vi "GetExternalInterfaces.vi"(8 "ErrorIn":errorcluster, 11 "ObjectIn":refnum<class "YAFTAF.lvclass">) -> (0 "ErrorOut":errorcluster, 2 "ExternalInterfaces":T1[](array[typedef]), 3 "ObjectOut":refnum<class "YAFTAF.lvclass">)   [LabVIEW 2021, in "YAFTAF.lvclass"]
uses:
  YAFTAF.lvclass
  C:/Localdata/Projects/TriekselSoft/TriekselsoftApplicationFramework/Source/.Externals/Library_YAF/YActor/YActor.lvclass
  Library_TAF_Support/ClusterArrayConversion/BundledArray.ctl
  YActor/YActor.lvclass/YActor.ctl
  YActor/ExeCmd_sync.vi
  YActor/private/SendCommand.vi
  YActor/private/WaitForReply.vi
  YActor/private/CreateLocalVI.vi
  YActor/private/ExeuteInlineVI.vi
  YActor/private/GetRemoteVIRef.vi
  YActor/private/GetNameOfVI.vi
  YActor/QuickCast.vi
  YActor/private/VINameProperty.vi
  YActor/private/MessageCounter.vi
  YActor/InlineReferencePool.vi
  YActor/private/ExecuteVI.vi
  YActor/YActor.lvclass
  YAFTAF.lvclass/YAFTAF.ctl
  Library_TAF_Support/ClusterArrayConversion/ClusterArrayConversion.lvlib
  C:/Localdata/Projects/TriekselSoft/TriekselsoftApplicationFramework/Source/.Externals/Interface_UserInterface_IFrontPanel/IFrontPanel/IFrontPanel.lvclass
  C:/Localdata/Projects/TriekselSoft/TriekselsoftApplicationFramework/Source/IInterface/IInterface.lvclass
  C:/Localdata/Projects/TriekselSoft/TriekselsoftApplicationFramework/Source/.Externals/Interface_Object_ICreateDestroy/ICreateDestroy/ICreateDestroy.lvclass
  C:/Localdata/Projects/TriekselSoft/TriekselsoftApplicationFramework/Source/.Externals/Interface_Object_IPersistentData/IPersistentData/IPersistentData.lvclass
  C:/Localdata/Projects/TriekselSoft/TriekselsoftApplicationFramework/Source/.Externals/Interface_TAF_ITAFObject/ITAFObject/ITAFObject.lvclass
  C:/Localdata/Projects/TriekselSoft/TriekselsoftApplicationFramework/Source/.Externals/Library_YAF/YAFTAF/YAFTAF.lvclass
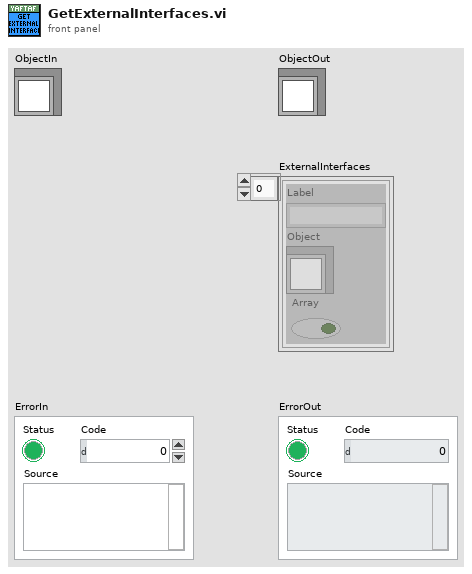
[diagram p1: front panel]
types:
  T1 = typedef "ClusterArrayConversion.lvlib/BundledArray.ctl" = cluster{"Label":string, "Object":refnum<class>, "Array":bool}
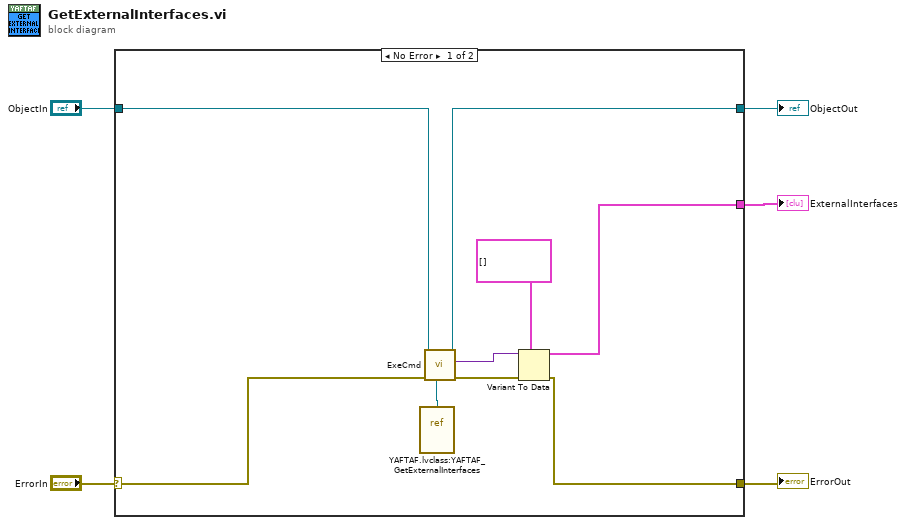
[diagram p0: block diagram]
diagram:
  n1 = case shown="No Error" "ErrorIn" {
    selector: "ErrorIn" -> [w12 w16]
    tunnel: [w13 w16] -> w4
    tunnel: [w8 w15] -> w2
    tunnel: "ObjectIn" -> [w7 w15]
    tunnel: [w6 _] -> w1
    frame No Error {
      n2 = vi-ref "YAFTAF.lvclass:YAFTAF_GetExternalInterfaces.vi"() -> (w11:refnum<vi>)
      n3 = call-poly "ExeCmd.vi"("CmdVIRef"=w11, "ErrorIn"=w12, "YActorIn"=w7) -> ("ErrorOut"=w14:errorcluster, "ReplyData"=w9:variant, "YActorOut"=w8:refnum<class "YAFTAF.lvclass">)  [unwired: 6 in]
      n4 = Variant To Data(error in=w14, type=T1[] [] ("ExternalInterfaces"), Variant=w9) -> (data=w6:T1[], error out=w13:errorcluster)
    }
    frame Error {
    }
  }
  "ErrorOut" <- w4
  "ObjectOut" <- w2
  "ExternalInterfaces" <- w1
